vi "JSONToSensorConfig.vi"(8 "ErrorIn":errorcluster, 11 "JSONIn":refnum<class "JSON Value.lvclass">) -> (0 "ErrorOut":errorcluster, 2 "SensorConfiguration":T1={"AccelFSRange"=enum."2G", "GyroFSRange"=enum."250DPS", "ODR"=enum."10HZ", "AccelDLPF"=enum."5HZ", "GyroDLPF"=enum."5HZ", "InterruptPinMode"=enum."OPEN_DRAIN_FALLING_EDGE", "InterruptMode"=enum."DATA_RDY", "Resolution"=4} {"Resolution" min=4 max=16 step=1}, 3 "JSONOut":refnum<class "JSON Value.lvclass">)   [LabVIEW 2016]
uses:
  <vilib>/addons/JSON API/JSON Value/JSON Value.lvclass
  FallSensor/ConfigureDevice/CDSensorConfiguration.ctl
  FallSensor/ConfigureDevice/CDAccelFSRange.ctl
  FallSensor/ConfigureDevice/CDGyroFSRange.ctl
  FallSensor/ConfigureDevice/CDOutputDataRate.ctl
  FallSensor/ConfigureDevice/CDAccelDLPF.ctl
  FallSensor/ConfigureDevice/CDGyroDLPF.ctl
  FallSensor/ConfigureDevice/CDInterruptPinMode.ctl
  FallSensor/ConfigureDevice/CDInterruptMode.ctl
  <vilib>/addons/JSON API/JSON Value/Get Object Item by Name.vi
  <vilib>/addons/JSON API/JSON Scalar/Get as Text.vi
  <vilib>/addons/JSON API/JSON Scalar/Get as U32.vi
  <vilib>/addons/JSON API/Get Polymorphic/JSON GetSet.lvlib
  <vilib>/addons/JSON API/JSON Scalar/JSON Scalar.lvclass
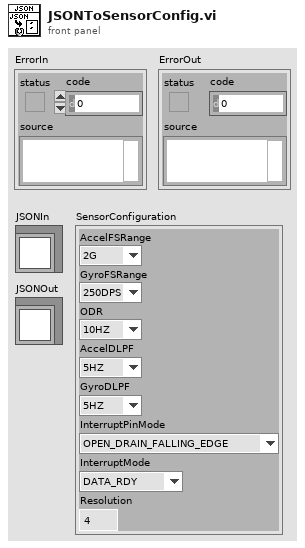
[diagram p1: front panel]
types:
  T1 = typedef "CDSensorConfiguration.ctl" = cluster{"AccelFSRange":T2, "GyroFSRange":T3, "ODR":T4, "AccelDLPF":T5, "GyroDLPF":T6, "InterruptPinMode":T7, "InterruptMode":T8, "Resolution":u32}
  T2 = typedef "CDAccelFSRange.ctl" = enum16{"2G", "4G", "8G", "16G"}
  T3 = typedef "CDGyroFSRange.ctl" = enum16{"250DPS", "500DPS", "1000DPS", "2000DPS"}
  T4 = typedef "CDOutputDataRate.ctl" = enum16{"10HZ", "20HZ", "40HZ", "50HZ", "100HZ", "200HZ", "500HZ", "1000HZ"}
  T5 = typedef "CDAccelDLPF.ctl" = enum16{"5HZ", "10HZ", "20HZ", "41HZ", "92HZ", "184HZ", "460HZ"}
  T6 = typedef "CDGyroDLPF.ctl" = enum16{"5HZ", "10HZ", "20HZ", "41HZ", "92HZ", "184HZ"}
  T7 = typedef "CDInterruptPinMode.ctl" = enum16{"OPEN_DRAIN_FALLING_EDGE"}
  T8 = typedef "CDInterruptMode.ctl" = enum16{"DATA_RDY"}
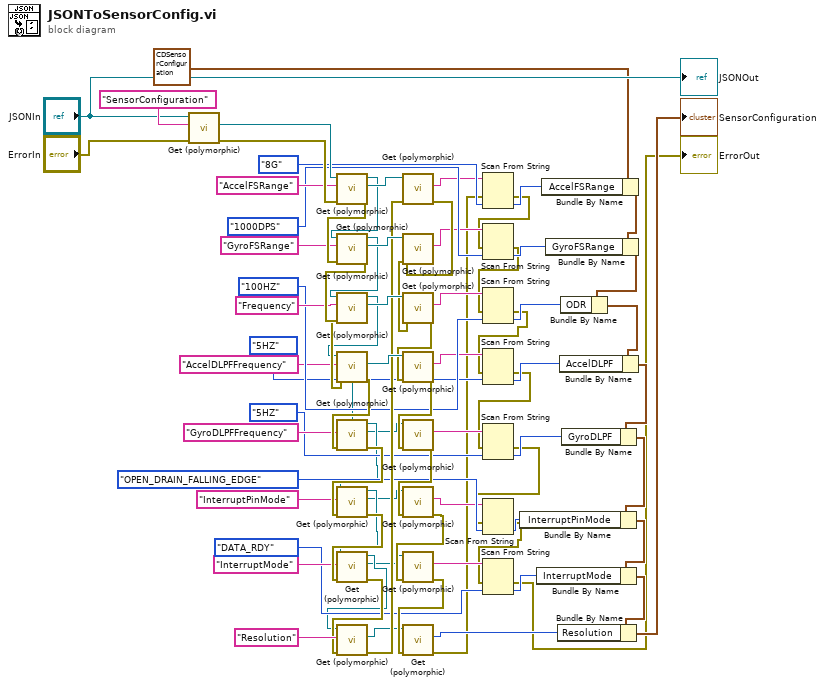
[diagram p0: block diagram]
diagram:
  n1 = call-poly <vilib>:"Get (polymorphic).vi"("error in (no error)"="ErrorIn", "name"="SensorConfiguration", "JSON Value In"="JSONIn") -> ("error out"=w67:errorcluster, "Value"=w66:refnum<class "JSON Value.lvclass">)  [unwired: 5 in, 2 out]
  n2 = call-poly <vilib>:"Get (polymorphic).vi"("error in (no error)"=w67, "name"="AccelFSRange", "JSON Value In"=w66) -> ("error out"=w77:errorcluster, "Value"=w82:refnum<class "JSON Value.lvclass">, "JSON Value Out"=w81:refnum<class "JSON Value.lvclass">)  [unwired: 5 in, 1 out]
  n3 = call-poly <vilib>:"Get (polymorphic).vi"("error in (no error)"=w77, "name"="GyroFSRange", "JSON Value In"=w81) -> ("error out"=w76:errorcluster, "Value"=w80:refnum<class "JSON Value.lvclass">, "JSON Value Out"=w79:refnum<class "JSON Value.lvclass">)  [unwired: 5 in, 1 out]
  n4 = call-poly <vilib>:"Get (polymorphic).vi"("error in (no error)"=w76, "name"="Frequency", "JSON Value In"=w79) -> ("error out"=w72:errorcluster, "Value"=w78:refnum<class "JSON Value.lvclass">, "JSON Value Out"=w70:refnum<class "JSON Value.lvclass">)  [unwired: 5 in, 1 out]
  n5 = call-poly <vilib>:"Get (polymorphic).vi"("error in (no error)"=w72, "name"="AccelDLPFFrequency", "JSON Value In"=w70) -> ("error out"=w61:errorcluster, "Value"=w71:refnum<class "JSON Value.lvclass">, "JSON Value Out"=w23:refnum<class "JSON Value.lvclass">)  [unwired: 5 in, 1 out]
  n6 = call-poly <vilib>:"Get (polymorphic).vi"("error in (no error)"=w61, "name"="GyroDLPFFrequency", "JSON Value In"=w23) -> ("error out"=w59:errorcluster, "Value"=w19:refnum<class "JSON Value.lvclass">, "JSON Value Out"=w22:refnum<class "JSON Value.lvclass">)  [unwired: 5 in, 1 out]
  n7 = call-poly <vilib>:"Get (polymorphic).vi"("error in (no error)"=w59, "name"="InterruptPinMode", "JSON Value In"=w22) -> ("error out"=w58:errorcluster, "Value"=w18:refnum<class "JSON Value.lvclass">, "JSON Value Out"=w21:refnum<class "JSON Value.lvclass">)  [unwired: 5 in, 1 out]
  n8 = call-poly <vilib>:"Get (polymorphic).vi"("error in (no error)"=w58, "name"="InterruptMode", "JSON Value In"=w21) -> ("error out"=w57:errorcluster, "Value"=w17:refnum<class "JSON Value.lvclass">, "JSON Value Out"=w20:refnum<class "JSON Value.lvclass">)  [unwired: 5 in, 1 out]
  n9 = call-poly <vilib>:"Get (polymorphic).vi"("error in (no error)"=w57, "name"="Resolution", "JSON Value In"=w20) -> ("error out"=w56:errorcluster, "Value"=w16:refnum<class "JSON Value.lvclass">)  [unwired: 5 in, 2 out]
  n10 = call-poly <vilib>:"Get (polymorphic).vi"("error in (no error)"=w56, "JSON Scalar in"=w82) -> ("error out"=w75:errorcluster, "LabVIEW Text"=w15:string)  [unwired: 7 in, 1 out]
  n11 = call-poly <vilib>:"Get (polymorphic).vi"("error in (no error)"=w75, "JSON Scalar in"=w80) -> ("error out"=w74:errorcluster, "LabVIEW Text"=w14:string)  [unwired: 7 in, 1 out]
  n12 = call-poly <vilib>:"Get (polymorphic).vi"("error in (no error)"=w74, "JSON Scalar in"=w78) -> ("error out"=w55:errorcluster, "LabVIEW Text"=w13:string)  [unwired: 7 in, 1 out]
  n13 = call-poly <vilib>:"Get (polymorphic).vi"("error in (no error)"=w55, "JSON Scalar in"=w71) -> ("error out"=w54:errorcluster, "LabVIEW Text"=w12:string)  [unwired: 7 in, 1 out]
  n14 = call-poly <vilib>:"Get (polymorphic).vi"("error in (no error)"=w54, "JSON Scalar in"=w19) -> ("error out"=w53:errorcluster, "LabVIEW Text"=w11:string)  [unwired: 7 in, 1 out]
  n15 = call-poly <vilib>:"Get (polymorphic).vi"("error in (no error)"=w53, "JSON Scalar in"=w18) -> ("error out"=w52:errorcluster, "LabVIEW Text"=w10:string)  [unwired: 7 in, 1 out]
  n16 = call-poly <vilib>:"Get (polymorphic).vi"("error in (no error)"=w52, "JSON Scalar in"=w17) -> ("error out"=w51:errorcluster, "LabVIEW Text"=w9:string)  [unwired: 7 in, 1 out]
  n17 = call-poly <vilib>:"Get (polymorphic).vi"("error in (no error)"=w51, "JSON Scalar in"=w16) -> ("error out"=w8:errorcluster, "Number"=w27:u32)  [unwired: 7 in, 1 out]
  n18 = Scan From String(input string=w15, error in=w8, default 1=CDAccelFSRange."8G" ("AccelFSRange")) -> (error out=w7:errorcluster, output 1=w48:T2)  [unwired: 2 in, 2 out]
  n19 = Scan From String(input string=w14, error in=w7, default 1=CDGyroFSRange."1000DPS" ("GyroFSRange")) -> (error out=w6:errorcluster, output 1=w42:T3)  [unwired: 2 in, 2 out]
  n20 = Scan From String(input string=w13, error in=w6, default 1=CDOutputDataRate."100HZ" ("ODR")) -> (error out=w5:errorcluster, output 1=w43:T4)  [unwired: 2 in, 2 out]
  n21 = Scan From String(input string=w12, error in=w5, default 1=CDAccelDLPF."5HZ" ("AccelDLPF")) -> (error out=w4:errorcluster, output 1=w39:T5)  [unwired: 2 in, 2 out]
  n22 = Scan From String(input string=w11, error in=w4, default 1=CDGyroDLPF."5HZ" ("GyroDLPF")) -> (error out=w3:errorcluster, output 1=w33:T6)  [unwired: 2 in, 2 out]
  n23 = Scan From String(input string=w10, error in=w3, default 1=CDInterruptPinMode."OPEN_DRAIN_FALLING_EDGE" ("InterruptPinMode")) -> (error out=w2:errorcluster, output 1=w34:T7)  [unwired: 2 in, 2 out]
  n24 = Scan From String(input string=w9, error in=w2, default 1=CDInterruptMode."DATA_RDY" ("InterruptMode")) -> (error out=→"ErrorOut":errorcluster, output 1=w24:T8)  [unwired: 2 in, 2 out]
  n25 = Bundle By Name(cluster=T1 {"AccelFSRange"=enum."2G", "GyroFSRange"=enum."250DPS", "ODR"=enum."10HZ", "AccelDLPF"=enum."5HZ", "GyroDLPF"=enum."5HZ", "InterruptPinMode"=enum."OPEN_DRAIN_FALLING_EDGE", "InterruptMode"=enum."DATA_RDY", "Resolution"=4} ("SensorConfiguration"), "AccelFSRange"=w48) -> (w73:T1)
  n26 = Bundle By Name(cluster=w73, "GyroFSRange"=w42) -> (w69:T1)
  n27 = Bundle By Name(cluster=w69, "ODR"=w43) -> (w62:T1)
  n28 = Bundle By Name(cluster=w62, "AccelDLPF"=w39) -> (w32:T1)
  n29 = Bundle By Name(cluster=w32, "GyroDLPF"=w33) -> (w28:T1)
  n30 = Bundle By Name(cluster=w28, "InterruptPinMode"=w34) -> (w31:T1)
  n31 = Bundle By Name(cluster=w31, "InterruptMode"=w24) -> (w30:T1)
  n32 = Bundle By Name(cluster=w30, "Resolution"=w27) -> (→"SensorConfiguration":T1)
  "JSONOut" <- "JSONIn"
